vi "Rate scan Find Offset.vi"(0 "FtHander IN":u32, 1 "Sumador":u8, 2 "Max Recorido Dac":i32=11, 4 "Valor buscado scalers (5000)":u16, 5 "Error IN":errorcluster, 6 "Espera acceso USB":u32, 7 "T Ventana":u32 format="%x") -> (14 "FtHander OUT":u32, 15 "Todos los valores":T2, 16 "VALORES START-STOP":T1, 19 "Error OUT":errorcluster)   [LabVIEW 2019]
uses:
  ASIC.digital offset start-stop.ctl
panel:
  out "barrido":u8
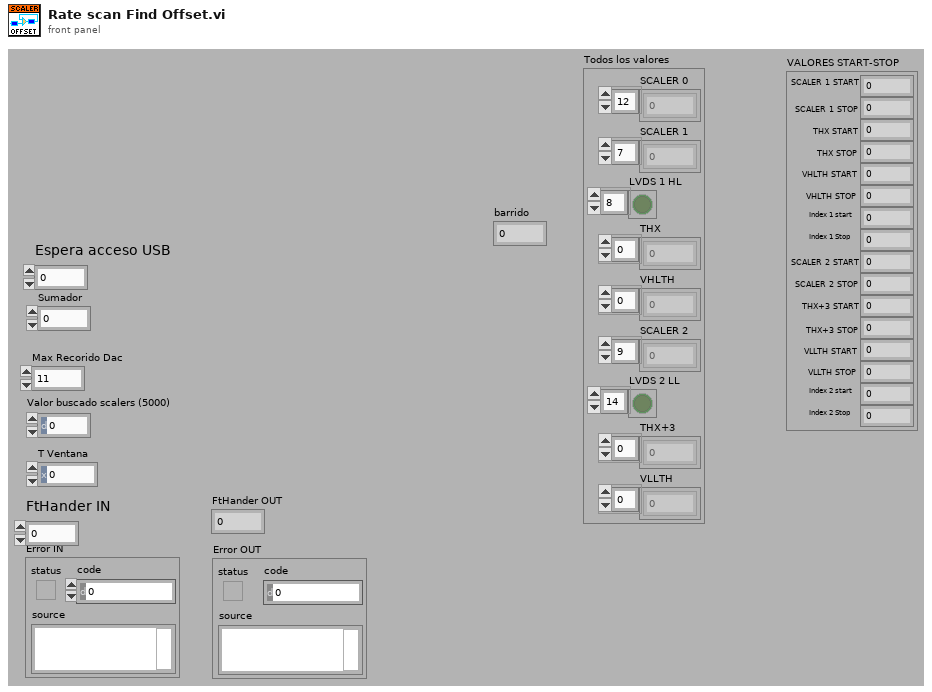
[diagram p1: front panel]
types:
  T1 = typedef "ASIC.digital offset start-stop.ctl" = cluster{"SCALER 1 START":u16, "SCALER 1 STOP":u16, "THX START":u16, "THX STOP":u16, "VHLTH START":dbl, "VHLTH STOP":dbl, "Index 1 start":i32, "Index 1 Stop":i32, "SCALER 2 START":u16, "SCALER 2 STOP":u16, "THX+3 START":u16, "THX+3 STOP":u16, "VLLTH START":dbl, "VLLTH STOP":dbl, "Index 2 start":i32, "Index 2 Stop":i32}
  T2 = cluster{"SCALER 0":u16[], "SCALER 1":u16[], "LVDS 1 HL":bool[], "THX":u16[], "VHLTH":dbl[], "SCALER 2":u16[], "LVDS 2 LL":bool[], "THX+3":u16[], "VLLTH":dbl[]}
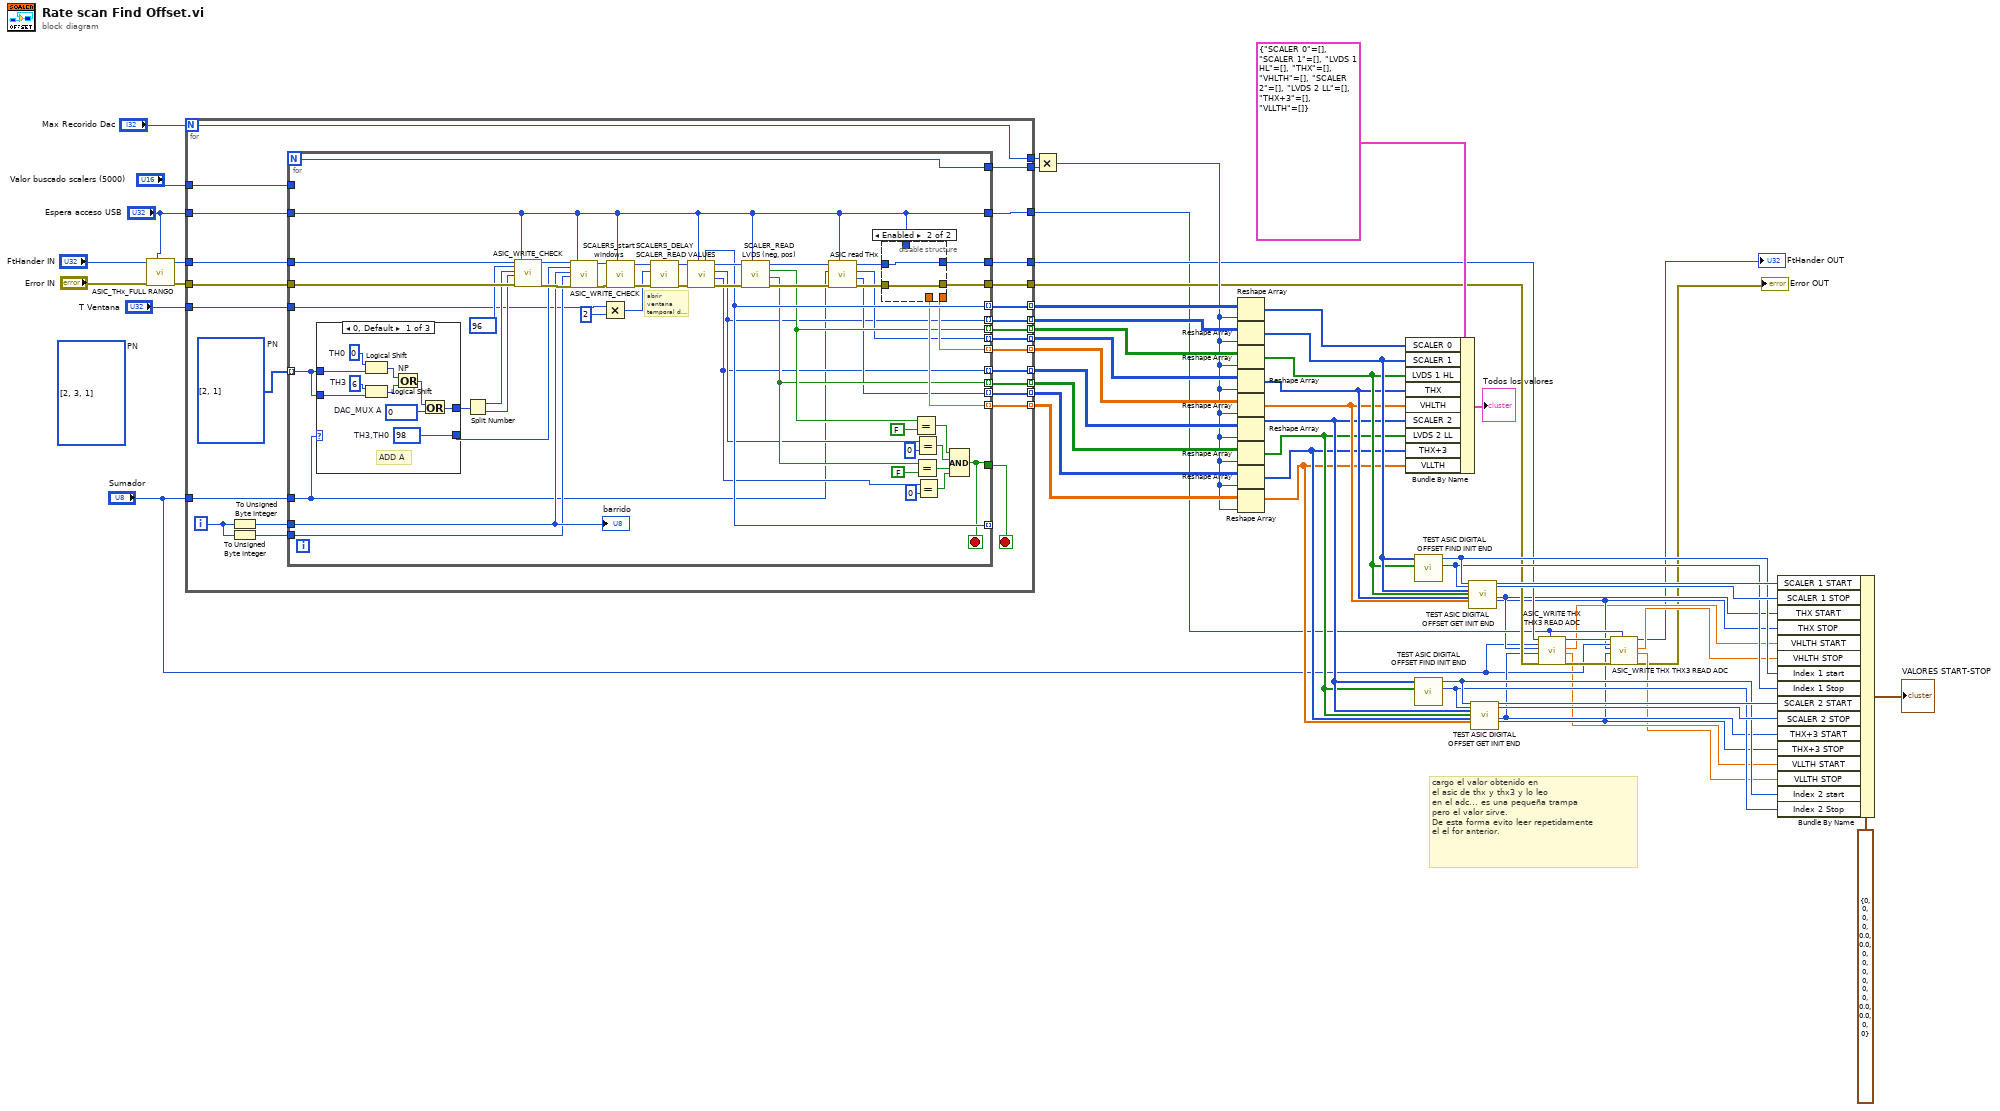
[diagram p0: block diagram]
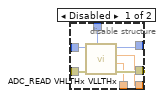
[diagram p2: hidden frame]
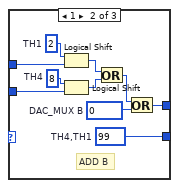
[diagram p3: hidden frame]
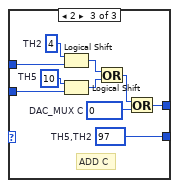
[diagram p4: hidden frame]
diagram:
  (unwired) u16[] [2, 3, 1]  # PN
  # "cargo el valor obtenido en\nel asic de thx y thx3 y lo leo\nen el adc... es una pequeña trampa\npero el valor sirve.\nDe esta forma evito leer repetidamente\nel el for anterior."
  n1 = call "ASIC_THx_FULL RANGO.vi"("Espera acceso USB"="Espera acceso USB", "error in"="Error IN", "ftHandle_in"="FtHander IN") -> ("error out"=w40:errorcluster, "ftHandle_out"=w41:u32)  [unwired: 7 in]
  n2 = for {
    N: "Max Recorido Dac" -> [w74]
    tunnel: "Espera acceso USB" -> [w62]
    tunnel: "T Ventana" -> [w82]
    tunnel: "Valor buscado scalers (5000)" -> [w75]
    tunnel: [w76] -> w14
    tunnel: [w74] -> w54
    tunnel: [w73] -> w53
    tunnel: [w72] -> w52 mode=indexing
    tunnel: [w71] -> w51 mode=indexing
    tunnel: [w70] -> w50 mode=indexing
    tunnel: [w69] -> w49 mode=indexing
    tunnel: [w68] -> w48 mode=indexing
    tunnel: [w67] -> w47 mode=indexing
    tunnel: [w66] -> w46 mode=indexing
    tunnel: [w65] -> w45 mode=indexing
    tunnel: [w64] -> w44 mode=indexing
    tunnel: "Sumador" -> [w58]
    tunnel: w41 -> [w61]
    tunnel: [w79] -> w16
    tunnel: w40 -> [w60]
    tunnel: [w78] -> w15
    i -> [w77]
    stop <- w63 stop-if-true
    w59 = u16[] [2, 1]  # PN
    n3 = To Unsigned Byte Integer(number=w77) -> (unsigned 8bit integer=w81:u8)
    n4 = To Unsigned Byte Integer(number=w77) -> (unsigned 8bit integer=w80:u8)
    n5 = for {
      N -> [w103]
      tunnel: w82 -> [w114]
      tunnel: w81 -> [w119]
      tunnel: w80 -> [w118]
      tunnel: w62 -> [w106]
      tunnel: w59 -> [w116] mode=indexing
      tunnel: [w106] -> w76
      tunnel: w75 -> [_]
      tunnel: [w102] -> _ mode=indexing
      tunnel: [w103] -> w73
      tunnel: [w102] -> w72 mode=indexing
      tunnel: [w86] -> w71 mode=indexing
      tunnel: [w99] -> w70 mode=indexing
      tunnel: [w97] -> w69 mode=indexing
      tunnel: [w101] -> w68 mode=indexing
      tunnel: [w85] -> w67 mode=indexing
      tunnel: [w93] -> w66 mode=indexing
      tunnel: [w92] -> w65 mode=indexing
      tunnel: [w100] -> w64 mode=indexing
      tunnel: [w87] -> w63
      tunnel: w58 -> [w83]
      tunnel: w61 -> [w128]
      tunnel: [w112] -> w79
      tunnel: w60 -> [w127]
      tunnel: [w111] -> w78
      stop <- w87 stop-if-true
      # "abrir ventana temporal de los scalers"
      n6 = case shown="0, Default" w83 {
        tunnel: [w151 w161 w171] -> w120
        tunnel: w116 -> [w150 w160 w170]
        tunnel: w116 -> [w149 w159 w169]
        tunnel: [w143 w153 w163] -> w121
        frame 0, Default {
          w142 = u16 0  # DAC_MUX A
          w147 = i8 6  # TH3
          w148 = i8 0  # TH0
          w151 = u8 98  # TH3,TH0
          # "ADD A"
          n7 = Logical Shift(y=w148, x=w150) -> (x << y=w145:u16)
          n8 = Logical Shift(y=w147, x=w149) -> (x << y=w146:u16)
          n9 = Or "NP"(x=w145, y=w146) -> (x .or. y?=w144:u16)
          n10 = Or(x=w144, y=w142) -> (x .or. y?=w143:u16)
        }
        frame 1 {
          w152 = u16 0  # DAC_MUX B
          w157 = i8 8  # TH4
          w158 = i8 2  # TH1
          w161 = u8 99  # TH4,TH1
          # "ADD B"
          n11 = Logical Shift(y=w158, x=w160) -> (x << y=w155:u16)
          n12 = Logical Shift(y=w157, x=w159) -> (x << y=w156:u16)
          n13 = Or(x=w155, y=w156) -> (x .or. y?=w154:u16)
          n14 = Or(x=w154, y=w152) -> (x .or. y?=w153:u16)
        }
        frame 2 {
          w162 = u16 0  # DAC_MUX C
          w167 = i8 10  # TH5
          w168 = i8 4  # TH2
          w171 = u8 97  # TH5,TH2
          # "ADD C"
          n15 = Logical Shift(y=w168, x=w170) -> (x << y=w165:u16)
          n16 = Logical Shift(y=w167, x=w169) -> (x << y=w166:u16)
          n17 = Or(x=w165, y=w166) -> (x .or. y?=w164:u16)
          n18 = Or(x=w164, y=w162) -> (x .or. y?=w163:u16)
        }
      }
      n19 = Split Number(x=w121) -> (hi(x)=w122:u8, lo(x)=w123:u8)
      n20 = call "ASIC_WRITE_CHECK.vi"("ftHandle_in"=w128, "Direccion Registro Asic"=u8 96, "Byte Alto"=w122, "Byte Bajo"=w123, "error in"=w127, "Espera acceso USB 2"=w106) -> ("ftHandle_out"=w125:u32, "error out"=w124:errorcluster)  [unwired: 11 in, 1 out]
      n21 = call "ASIC_WRITE_CHECK.vi"("ftHandle_in"=w125, "Direccion Registro Asic"=w120, "Byte Alto"=w119, "Byte Bajo"=w118, "error in"=w124, "Espera acceso USB 2"=w106) -> ("ftHandle_out"=w84:u32, "error out"=w117:errorcluster)  [unwired: 11 in, 1 out]
      n22 = Multiply(x=w114, y=u32 2) -> (x*y=w115:u32)
      n23 = call "SCALERS_start windows.vi"("Espera acceso USB"=w106, "error in 2"=w117, "ftHandle_in 2"=w84) -> ("error out"=w131:errorcluster, "ftHandle_out"=w132:u32)  [unwired: 7 in]
      n24 = call "SCALERS_DELAY.vi"("error out 2"=w131, "Ventana 2"=w115, "ftHandle_out 2"=w132) -> ("error out"=w129:errorcluster, "ftHandle_out"=w130:u32)  [unwired: 7 in]
      n25 = call "SCALER_READ VALUES.vi"("Espera acceso USB"=w106, "error in"=w129, "ftHandle_in"=w130) -> ("error out"=w108:errorcluster, "Scaler 3"=w85:u16, "Scaler 2"=w86:u16, "ftHandle_out"=w110:u32, "Scaler 1"=w102:u16)  [unwired: 3 in, 1 out]
      n26 = call "SCALER_READ LVDS (neg, pos).vi"("Espera acceso USB"=w106, "error in"=w108, "ftHandle_in"=w110) -> ("error out"=w107:errorcluster, "LVDS LLTH"=w93:bool, "LVDS HLTH"=w99:bool, "ftHandle_out"=w109:u32)  [unwired: 5 in]
      n27 = call "ASIC read THx.vi"("Espera acceso USB"=w106, "error in"=w107, "Sumador"=w83, "ftHandle_in"=w109) -> ("error out 2"=w104:errorcluster, "THx+3"=w92:u16, "THx"=w97:u16, "ftHandle_out 2"=w105:u32)  [unwired: 4 in]
      n28 = disable-structure shown="Enabled" {
        disable-tunnel: [w139 w141] -> w112
        disable-tunnel: [w138 w140] -> w111
        disable-tunnel: w106 -> [w137 _]
        disable-tunnel: w105 -> [w136 w141]
        disable-tunnel: w104 -> [w135 w140]
        disable-tunnel: [w134 _] -> w101
        disable-tunnel: [w133 _] -> w100
        frame Disabled {
          n29 = call "ADC_READ VHLTHx VLLTHx.vi"("Espera acceso FT"=w137, "error out 2"=w135, "ftHandle_out 2"=w136) -> ("error out"=w138:errorcluster, "LLTHx"=w133:dbl, "HLTHx"=w134:dbl, "ftHandle_out"=w139:u32)  [unwired: 5 in]
        }
        frame Enabled {
        }
      }
      n30 = Equal?(x=w99, y=FALSE) -> (x = y?=w91:bool)
      n31 = Equal?(x=w93, y=FALSE) -> (x = y?=w89:bool)
      n32 = Equal?(x=w86, y=u16 0) -> (x = y?=w90:bool)
      n33 = Equal?(x=w85, y=u16 0) -> (x = y?=w88:bool)
      n34 = Compound Arithmetic op=AND(w91, w90, w89, w88) -> (w87:bool)
      "barrido" <- w119
    }
  }
  n35 = Multiply(x=w54, y=w53) -> (x*y=w43:i32)
  n36 = Reshape Array(w52, w43) -> (w38:u16[])
  n37 = Reshape Array(w51, w43) -> (w37:u16[])
  n38 = Reshape Array(w50, w43) -> (w36:bool[])
  n39 = Reshape Array(w49, w43) -> (w35:u16[])
  n40 = Reshape Array(w48, w43) -> (w34:dbl[])
  n41 = Reshape Array(w47, w43) -> (w33:u16[])
  n42 = Reshape Array(w46, w43) -> (w32:bool[])
  n43 = Reshape Array(w45, w43) -> (w31:u16[])
  n44 = Reshape Array(w44, w43) -> (w30:dbl[])
  n45 = Bundle By Name(cluster=T2 {"SCALER 0"=[], "SCALER 1"=[], "LVDS 1 HL"=[], "THX"=[], "VHLTH"=[], "SCALER 2"=[], "LVDS 2 LL"=[], "THX+3"=[], "VLLTH"=[]}, "SCALER 0"=w38, "SCALER 1"=w37, "LVDS 1 HL"=w36, "THX"=w35, "VHLTH"=w34, "SCALER 2"=w33, "LVDS 2 LL"=w32, "THX+3"=w31, "VLLTH"=w30) -> (→"Todos los valores":T2)
  n46 = call "TEST ASIC DIGITAL OFFSET FIND INIT END.vi"("LVDS"=w36, "SCALER"=w37) -> ("Max"=w22:i32, "Min"=w23:i32)  [unwired: 8 in]
  n47 = call "TEST ASIC DIGITAL OFFSET FIND INIT END.vi"("LVDS"=w32, "SCALER"=w33) -> ("Max"=w20:i32, "Min"=w21:i32)  [unwired: 8 in]
  n48 = call "TEST ASIC DIGITAL OFFSET GET INIT END.vi"("Min"=w23, "Max"=w22, "Scaler x"=w37, "LVDS x"=w36, "THx"=w35, "VxLTH"=w34) -> ("Scaler X min"=w28:u16, "Scaler X Max"=w27:u16, "THX min"=w11:u16, "THX Max"=w7:u16)  [unwired: 14 in, 4 out]
  n49 = call "TEST ASIC DIGITAL OFFSET GET INIT END.vi"("Min"=w21, "Max"=w20, "Scaler x"=w33, "LVDS x"=w32, "THx"=w31, "VxLTH"=w30) -> ("Scaler X min"=w24:u16, "Scaler X Max"=w26:u16, "THX min"=w10:u16, "THX Max"=w8:u16)  [unwired: 14 in, 4 out]
  n50 = call "ASIC_WRITE THX THX3 READ ADC.vi"("ftHandle_in"=w16, "Sumador"="Sumador", "THX"=w11, "THX+3"=w10, "error in"=w15, "Espera acceso USB 2"=w14) -> ("ftHandle_out"=w13:u32, "HLTHx"=w6:dbl, "LLTHx"=w5:dbl, "error out"=w12:errorcluster)  [unwired: 10 in]
  n51 = call "ASIC_WRITE THX THX3 READ ADC.vi"("ftHandle_in"=w13, "Sumador"="Sumador", "THX"=w7, "THX+3"=w8, "error in"=w12, "Espera acceso USB 2"=w14) -> ("ftHandle_out"=→"FtHander OUT":u32, "HLTHx"=w4:dbl, "LLTHx"=w3:dbl, "error out"=→"Error OUT":errorcluster)  [unwired: 10 in]
  n52 = Bundle By Name(cluster=T1 {"SCALER 1 START"=0, "SCALER 1 STOP"=0, "THX START"=0, "THX STOP"=0, "VHLTH START"=0.0, "VHLTH STOP"=0.0, "Index 1 start"=0, "Index 1 Stop"=0, "SCALER 2 START"=0, "SCALER 2 STOP"=0, "THX+3 START"=0, "THX+3 STOP"=0, "VLLTH START"=0.0, "VLLTH STOP"=0.0, "Index 2 start"=0, "Index 2 Stop"=0}, "SCALER 1 START"=w28, "SCALER 1 STOP"=w27, "THX START"=w11, "THX STOP"=w7, "VHLTH START"=w6, "VHLTH STOP"=w4, "Index 1 start"=w23, "Index 1 Stop"=w22, "SCALER 2 START"=w24, "SCALER 2 STOP"=w26, "THX+3 START"=w10, "THX+3 STOP"=w8, "VLLTH START"=w5, "VLLTH STOP"=w3, "Index 2 start"=w21, "Index 2 Stop"=w20) -> (→"VALORES START-STOP":T1)
